vi "getPublications_Reply.vi"(9 "Topic Types":string[](array[string]), 11 "Published Topics":string[](array[string])) -> ()   [LabVIEW 2012]
panel:
  out "value":string
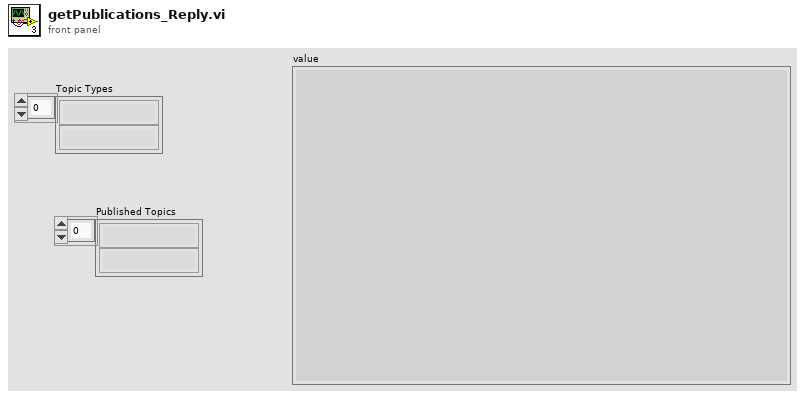
[diagram p1: front panel]
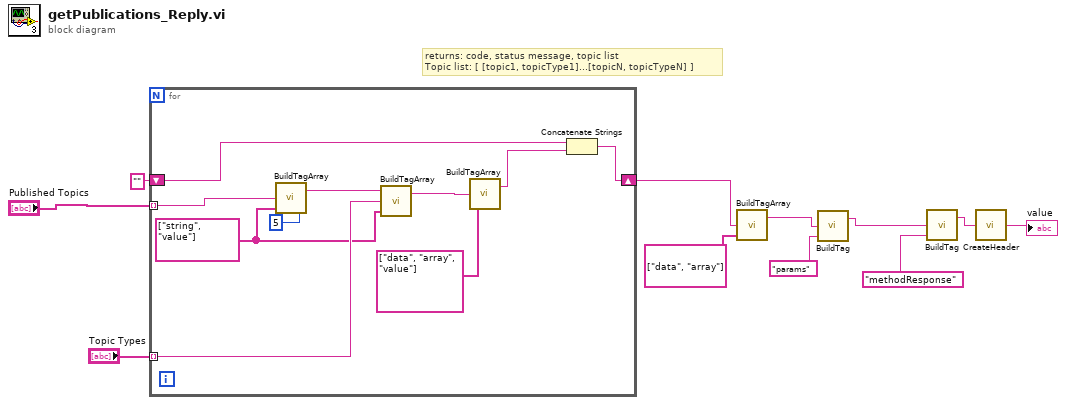
[diagram p0: block diagram]
diagram:
  # "returns: code, status message, topic list\nTopic list: [ [topic1, topicType1]...[topicN, topicTypeN] ]"
  n1 = for {
    tunnel: "Published Topics" -> [w21] mode=indexing
    tunnel: "Topic Types" -> [w19] mode=indexing
    shift-right: [w14] -> w7
    shift-left: "" ("value") -> [w15]
    w18 = string[] ["string", "value"] ("tags")
    n2 = call <userlib>:"BuildTagArray.vi"("Indent"=i8 5, "tags"=w18, "value"=w21) -> ("string out"=w20:string)  [unwired: 1 in]
    n3 = call <userlib>:"BuildTagArray.vi"("tags"=w18, "value"=w19, "string in"=w20) -> ("string out"=w17:string)  [unwired: 1 in]
    n4 = call <userlib>:"BuildTagArray.vi"("tags"=string[] ["data", "array", "value"], "value"=w17) -> ("string out"=w13:string)  [unwired: 2 in]
    n5 = Concatenate Strings(w15, w13) -> (w14:string)
  }
  n6 = call <userlib>:"BuildTagArray.vi"("tags"=string[] ["data", "array"], "value"=w7) -> ("string out"=w3:string)  [unwired: 2 in]
  n7 = call <userlib>:"BuildTag.vi"("tag"="params", "value"=w3) -> ("string out"=w1:string)  [unwired: 2 in]
  n8 = call <userlib>:"BuildTag.vi"("tag"="methodResponse", "value"=w1) -> ("string out"=w5:string)  [unwired: 2 in]
  n9 = call <userlib>:"CreateHeader.vi"("Content"=w5) -> ("XML"=→"value":string)
